vi "Set Position.vi"(8 "error in":errorcluster, 9 "Datum":T1, 10 "Target Coordinates":T2, 11 "Philips Dialog in":refnum<class "Flex UI Dialog.lvclass">) -> (0 "error out":errorcluster, 3 "Philips Dialog out":refnum<class "Flex UI Dialog.lvclass">)   [LabVIEW 2014, in "Flex UI Dialog.lvclass"]
doc: "Sets the position of the UI.\n\nThe Datum input specifies which part of the VI panel should be sent to those coordinates. For example, the Top-Left (corner) versus the Center point of the panel."
uses:
  Flex UI Dialog.lvclass
  <vilib>/Utility/miscctls.llb/LVPositionTypeDef.ctl
  Flex UI (Parent)/Enum - Datum.ctl
  Flex UI (Parent)/Flex UI.lvclass/Flex UI.ctl
  Flex UI (Parent)/Flex UI.lvclass
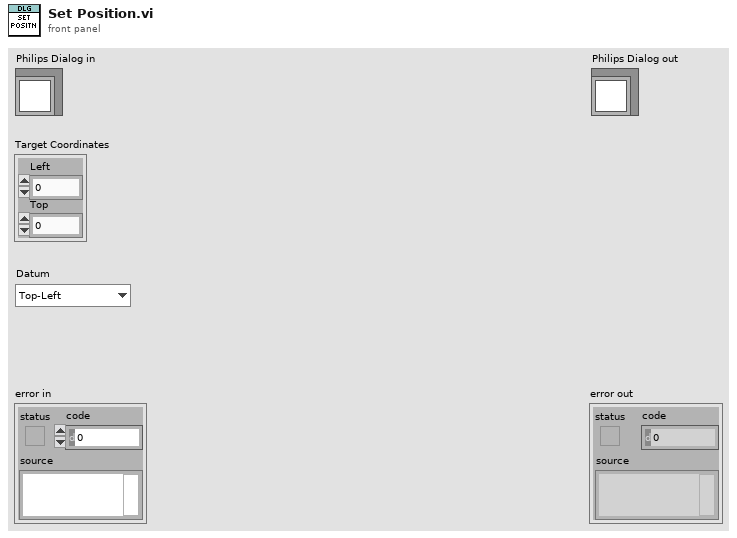
[diagram p1: front panel]
types:
  T1 = typedef "Flex UI.lvclass/Enum - Datum.ctl" = enum16{"Top-Left", "Top-Right", "Bottom-Left", "Bottom-Right", "Center"}
  T2 = typedef "LVPositionTypeDef.ctl" = cluster{"Left":i32, "Top":i32}
  T3 = typedef "LVRectTypeDef.ctl" = cluster{"Left":i16, "Top":i16, "Right":i16, "Bottom":i16}
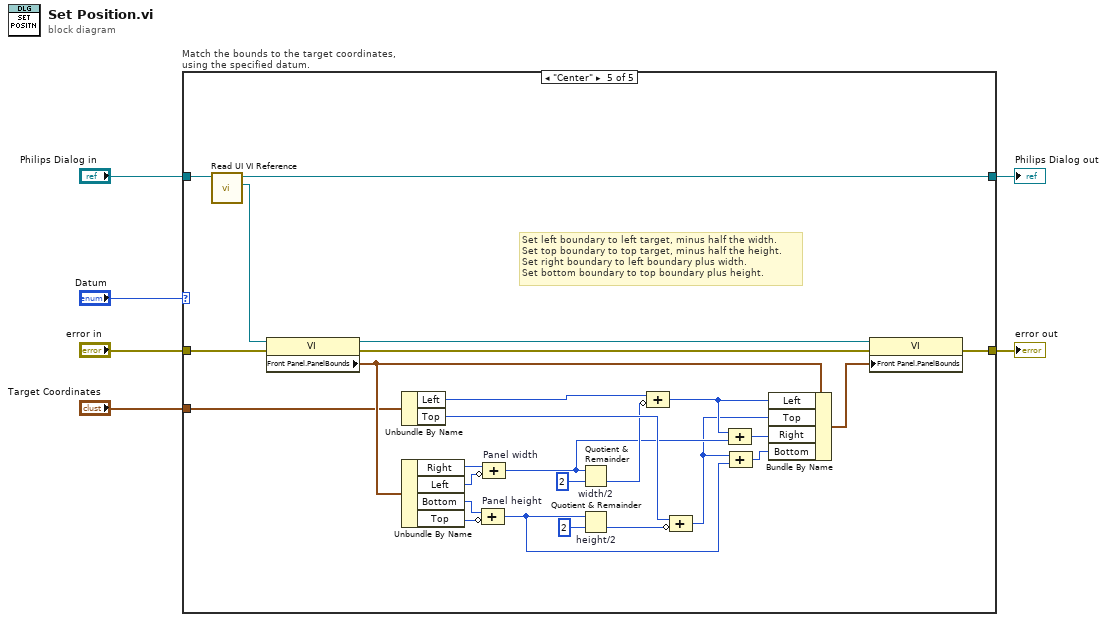
[diagram p0: block diagram]
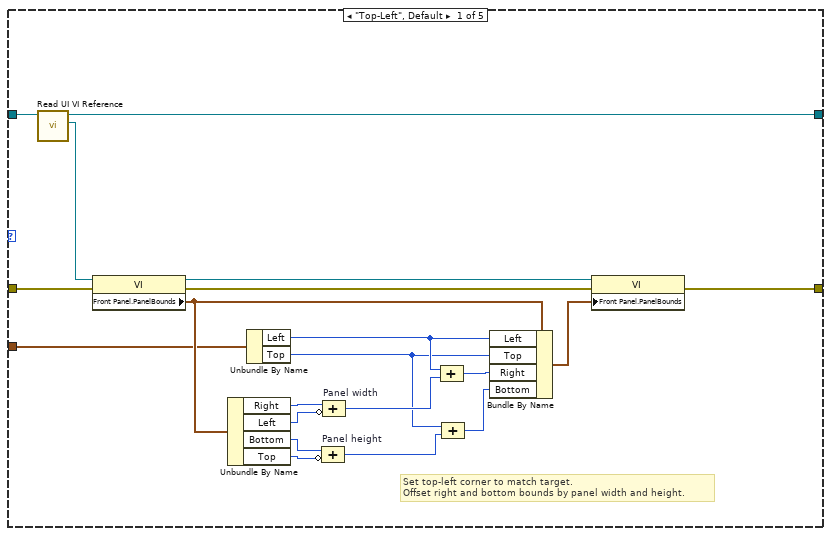
[diagram p2: hidden frame]
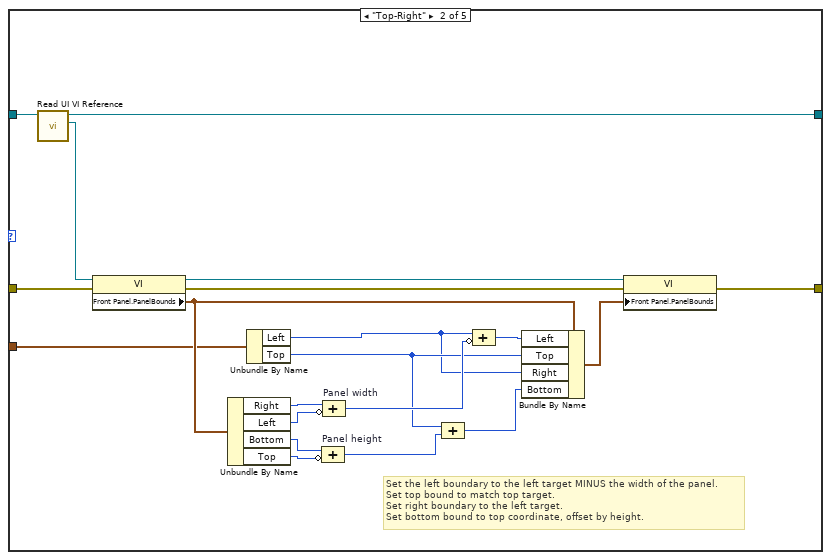
[diagram p3: hidden frame]
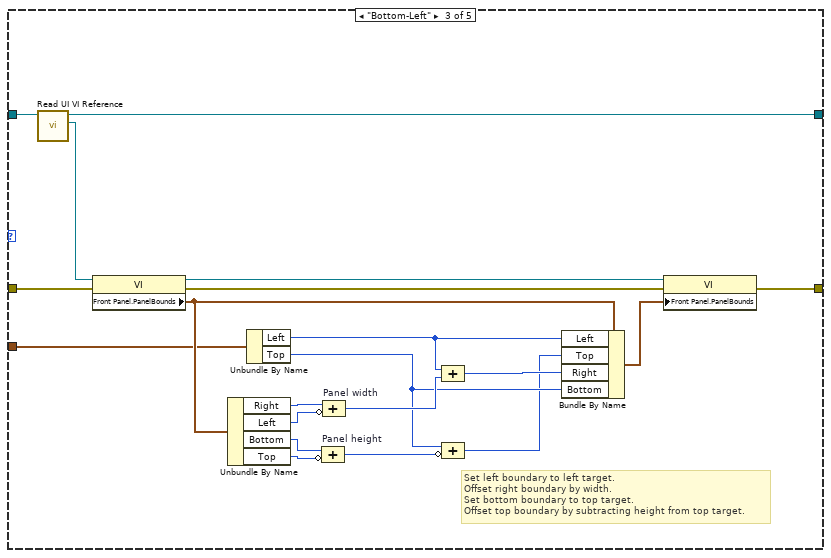
[diagram p4: hidden frame]
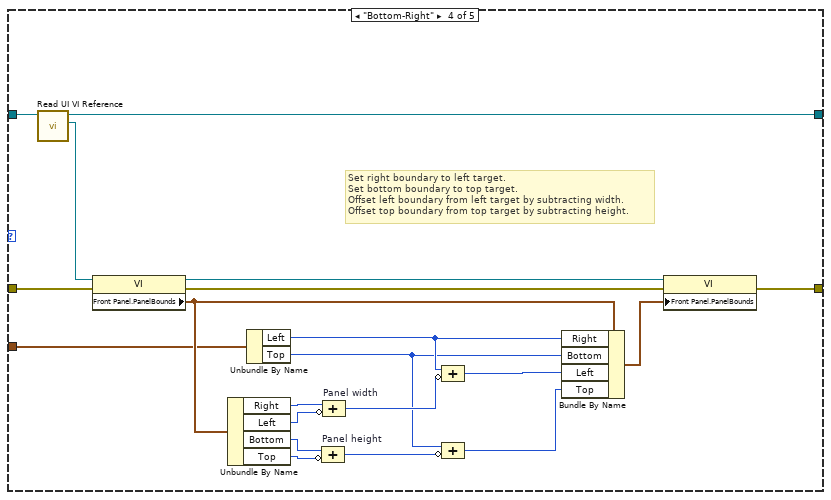
[diagram p5: hidden frame]
diagram:
  n1 = case "Match the bounds to the target coordinates, using the specified datum." shown="\"Center\"" "Datum" {
    tunnel: [w24 w44 w64 w84 w110] -> w5
    tunnel: "Philips Dialog in" -> [w25 w45 w65 w85 w111]
    tunnel: [w17 w37 w57 w77 w103] -> w3
    tunnel: "error in" -> [w26 w46 w66 w86 w112]
    tunnel: "Target Coordinates" -> [w14 w34 w54 w74 w100]
    frame "Top-Left", Default {
      # "Set top-left corner to match target.\nOffset right and bottom bounds by panel width and height."
      n2 = call "Read UI VI Reference.vi"("Philips UI in"=w25) -> ("UI VI Reference"=w22:refnum<vi>, "Philips UI out"=w24:refnum<class "Flex UI Dialog.lvclass">)  [unwired: 9 in]
      n3 = property class="VI"(reference=w22, error in=w26) -> (reference out=w16:refnum<vi>, error out=w23:errorcluster, "Front Panel.PanelBounds"=w15:T3)
      n4 = Unbundle By Name(w15) -> ("Right"=w21:i16, "Left"=w20:i16, "Bottom"=w19:i16, "Top"=w18:i16)
      n5 = Unbundle By Name(w14) -> ("Left"=w12:i32, "Top"=w9:i32)
      n6 = Compound Arithmetic op=ADD "Panel height"(w19, invert w18) -> (w8:i16)
      n7 = Compound Arithmetic op=ADD "Panel width"(w21, invert w20) -> (w13:i16)
      n8 = Compound Arithmetic op=ADD(w12, w13) -> (w11:i32)
      n9 = Compound Arithmetic op=ADD(w9, w8) -> (w7:i32)
      n10 = Bundle By Name(cluster=w15, "Left"=w12, "Top"=w9, "Right"=w11, "Bottom"=w7) -> (w10:T3)
      n11 = property class="VI"(reference=w16, error in=w23, "Front Panel.PanelBounds"=w10) -> (error out=w17:errorcluster)  [unwired: 1 out]
    }
    frame "Top-Right" {
      # "Set the left boundary to the left target MINUS the width of the panel.\nSet top bound to match top target.\nSet right boundary to the left target.\nSet bottom bound to top coordinate, offset by height."
      n12 = call "Read UI VI Reference.vi"("Philips UI in"=w45) -> ("UI VI Reference"=w42:refnum<vi>, "Philips UI out"=w44:refnum<class "Flex UI Dialog.lvclass">)  [unwired: 9 in]
      n13 = property class="VI"(reference=w42, error in=w46) -> (reference out=w36:refnum<vi>, error out=w43:errorcluster, "Front Panel.PanelBounds"=w35:T3)
      n14 = Unbundle By Name(w35) -> ("Right"=w41:i16, "Left"=w40:i16, "Bottom"=w39:i16, "Top"=w38:i16)
      n15 = Unbundle By Name(w34) -> ("Left"=w27:i32, "Top"=w31:i32)
      n16 = Compound Arithmetic op=ADD "Panel height"(w39, invert w38) -> (w30:i16)
      n17 = Compound Arithmetic op=ADD "Panel width"(w41, invert w40) -> (w33:i16)
      n18 = Compound Arithmetic op=ADD(w31, w30) -> (w29:i32)
      n19 = Compound Arithmetic op=ADD(w27, invert w33) -> (w28:i32)
      n20 = Bundle By Name(cluster=w35, "Left"=w28, "Top"=w31, "Right"=w27, "Bottom"=w29) -> (w32:T3)
      n21 = property class="VI"(reference=w36, error in=w43, "Front Panel.PanelBounds"=w32) -> (error out=w37:errorcluster)  [unwired: 1 out]
    }
    frame "Bottom-Left" {
      # "Set left boundary to left target.\nOffset right boundary by width.\nSet bottom boundary to top target.\nOffset top boundary by subtracting height from top target."
      n22 = call "Read UI VI Reference.vi"("Philips UI in"=w65) -> ("UI VI Reference"=w62:refnum<vi>, "Philips UI out"=w64:refnum<class "Flex UI Dialog.lvclass">)  [unwired: 9 in]
      n23 = property class="VI"(reference=w62, error in=w66) -> (reference out=w56:refnum<vi>, error out=w63:errorcluster, "Front Panel.PanelBounds"=w55:T3)
      n24 = Unbundle By Name(w55) -> ("Right"=w61:i16, "Left"=w60:i16, "Bottom"=w59:i16, "Top"=w58:i16)
      n25 = Unbundle By Name(w54) -> ("Left"=w51:i32, "Top"=w48:i32)
      n26 = Compound Arithmetic op=ADD "Panel height"(w59, invert w58) -> (w52:i16)
      n27 = Compound Arithmetic op=ADD "Panel width"(w61, invert w60) -> (w50:i16)
      n28 = Compound Arithmetic op=ADD(w51, w50) -> (w49:i32)
      n29 = Compound Arithmetic op=ADD(w48, invert w52) -> (w47:i32)
      n30 = Bundle By Name(cluster=w55, "Left"=w51, "Top"=w47, "Right"=w49, "Bottom"=w48) -> (w53:T3)
      n31 = property class="VI"(reference=w56, error in=w63, "Front Panel.PanelBounds"=w53) -> (error out=w57:errorcluster)  [unwired: 1 out]
    }
    frame "Bottom-Right" {
      # "Set right boundary to left target.\nSet bottom boundary to top target.\nOffset left boundary from left target by subtracting width.\nOffset top boundary from top target by subtracting height."
      n32 = call "Read UI VI Reference.vi"("Philips UI in"=w85) -> ("UI VI Reference"=w82:refnum<vi>, "Philips UI out"=w84:refnum<class "Flex UI Dialog.lvclass">)  [unwired: 9 in]
      n33 = property class="VI"(reference=w82, error in=w86) -> (reference out=w76:refnum<vi>, error out=w83:errorcluster, "Front Panel.PanelBounds"=w75:T3)
      n34 = Unbundle By Name(w75) -> ("Right"=w81:i16, "Left"=w80:i16, "Bottom"=w79:i16, "Top"=w78:i16)
      n35 = Unbundle By Name(w74) -> ("Left"=w70:i32, "Top"=w69:i32)
      n36 = Compound Arithmetic op=ADD "Panel height"(w79, invert w78) -> (w72:i16)
      n37 = Compound Arithmetic op=ADD "Panel width"(w81, invert w80) -> (w71:i16)
      n38 = Compound Arithmetic op=ADD(w70, invert w71) -> (w68:i32)
      n39 = Compound Arithmetic op=ADD(w69, invert w72) -> (w67:i32)
      n40 = Bundle By Name(cluster=w75, "Right"=w70, "Bottom"=w69, "Left"=w68, "Top"=w67) -> (w73:T3)
      n41 = property class="VI"(reference=w76, error in=w83, "Front Panel.PanelBounds"=w73) -> (error out=w77:errorcluster)  [unwired: 1 out]
    }
    frame "Center" {
      # "Set left boundary to left target, minus half the width.\nSet top boundary to top target, minus half the height.\nSet right boundary to left boundary plus width.\nSet bottom boundary to top boundary plus height."
      n42 = call "Read UI VI Reference.vi"("Philips UI in"=w111) -> ("UI VI Reference"=w108:refnum<vi>, "Philips UI out"=w110:refnum<class "Flex UI Dialog.lvclass">)  [unwired: 9 in]
      n43 = property class="VI"(reference=w108, error in=w112) -> (reference out=w102:refnum<vi>, error out=w109:errorcluster, "Front Panel.PanelBounds"=w101:T3)
      n44 = Unbundle By Name(w100) -> ("Left"=w98:i32, "Top"=w97:i32)
      n45 = Unbundle By Name(w101) -> ("Right"=w107:i16, "Left"=w106:i16, "Bottom"=w105:i16, "Top"=w104:i16)
      n46 = Compound Arithmetic op=ADD "Panel height"(w105, invert w104) -> (w87:i16)
      n47 = Compound Arithmetic op=ADD "Panel width"(w107, invert w106) -> (w91:i16)
      n48 = Quotient & Remainder "width/2"(x=w91, y=i16 2) -> (floor(x/y)=w95:i16)  [unwired: 1 out]
      n49 = Quotient & Remainder "height/2"(x=w87, y=i16 2) -> (floor(x/y)=w93:i16)  [unwired: 1 out]
      n50 = Compound Arithmetic op=ADD(w98, invert w95) -> (w92:i32)
      n51 = Compound Arithmetic op=ADD(w97, invert w93) -> (w89:i32)
      n52 = Compound Arithmetic op=ADD(w92, w91) -> (w90:i32)
      n53 = Compound Arithmetic op=ADD(w89, w87) -> (w88:i32)
      n54 = Bundle By Name(cluster=w101, "Left"=w92, "Top"=w89, "Right"=w90, "Bottom"=w88) -> (w99:T3)
      n55 = property class="VI"(reference=w102, error in=w109, "Front Panel.PanelBounds"=w99) -> (error out=w103:errorcluster)  [unwired: 1 out]
    }
  }
  "error out" <- w3
  "Philips Dialog out" <- w5
